vi "首页.vi"() -> ()   [LabVIEW 2016]
uses:
  <vilib>/Utility/miscctls.llb/LVPointTypeDef.ctl
  <vilib>/Utility/sysdir.llb/System Directory Type.ctl
  <vilib>/addons/database/_DB Variant To Data/Database Variant To Data.xnode
  PLC/PLC.lvlib
panel:
  out "小项目框 6":T1(xcontrol)
  out "小项目框 5":T1(xcontrol)
  out "小项目框":T1(xcontrol)
  out "湿度":string="75.5 %"
  out "室温":string="25.8 ℃"
  out "小项目框 4":T1(xcontrol)
  out "小项目框 3":T1(xcontrol)
  out "小项目框 2":T1(xcontrol)
  # "湿度:"
  # "室温:"
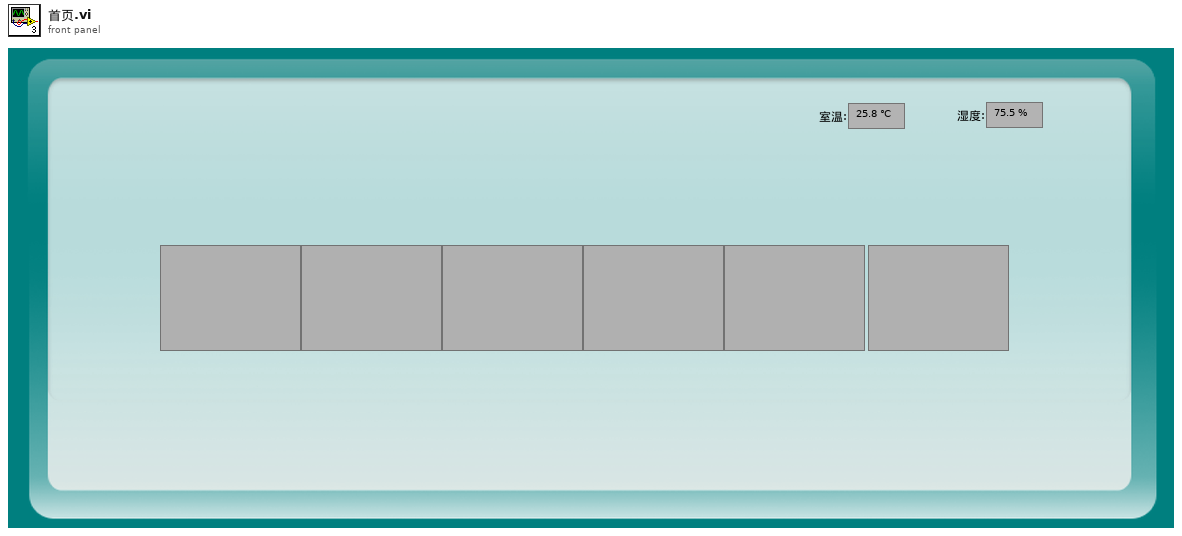
[diagram p1: front panel]
types:
  T1 = cluster{"中文项目名称":string, "英文项目名称":string, "单位":string, "浓度值":sgl}
  T2 = typedef "System Directory Type.ctl" = i32
  T3 = typedef "LVPointTypeDef.ctl" = cluster{"Horizontal":i16, "Vertical":i16}
  T4 = cluster{"AD0":sgl, "AD1":sgl, "AD2":sgl, "AD3":sgl, "AD4":sgl, "AD5":sgl}
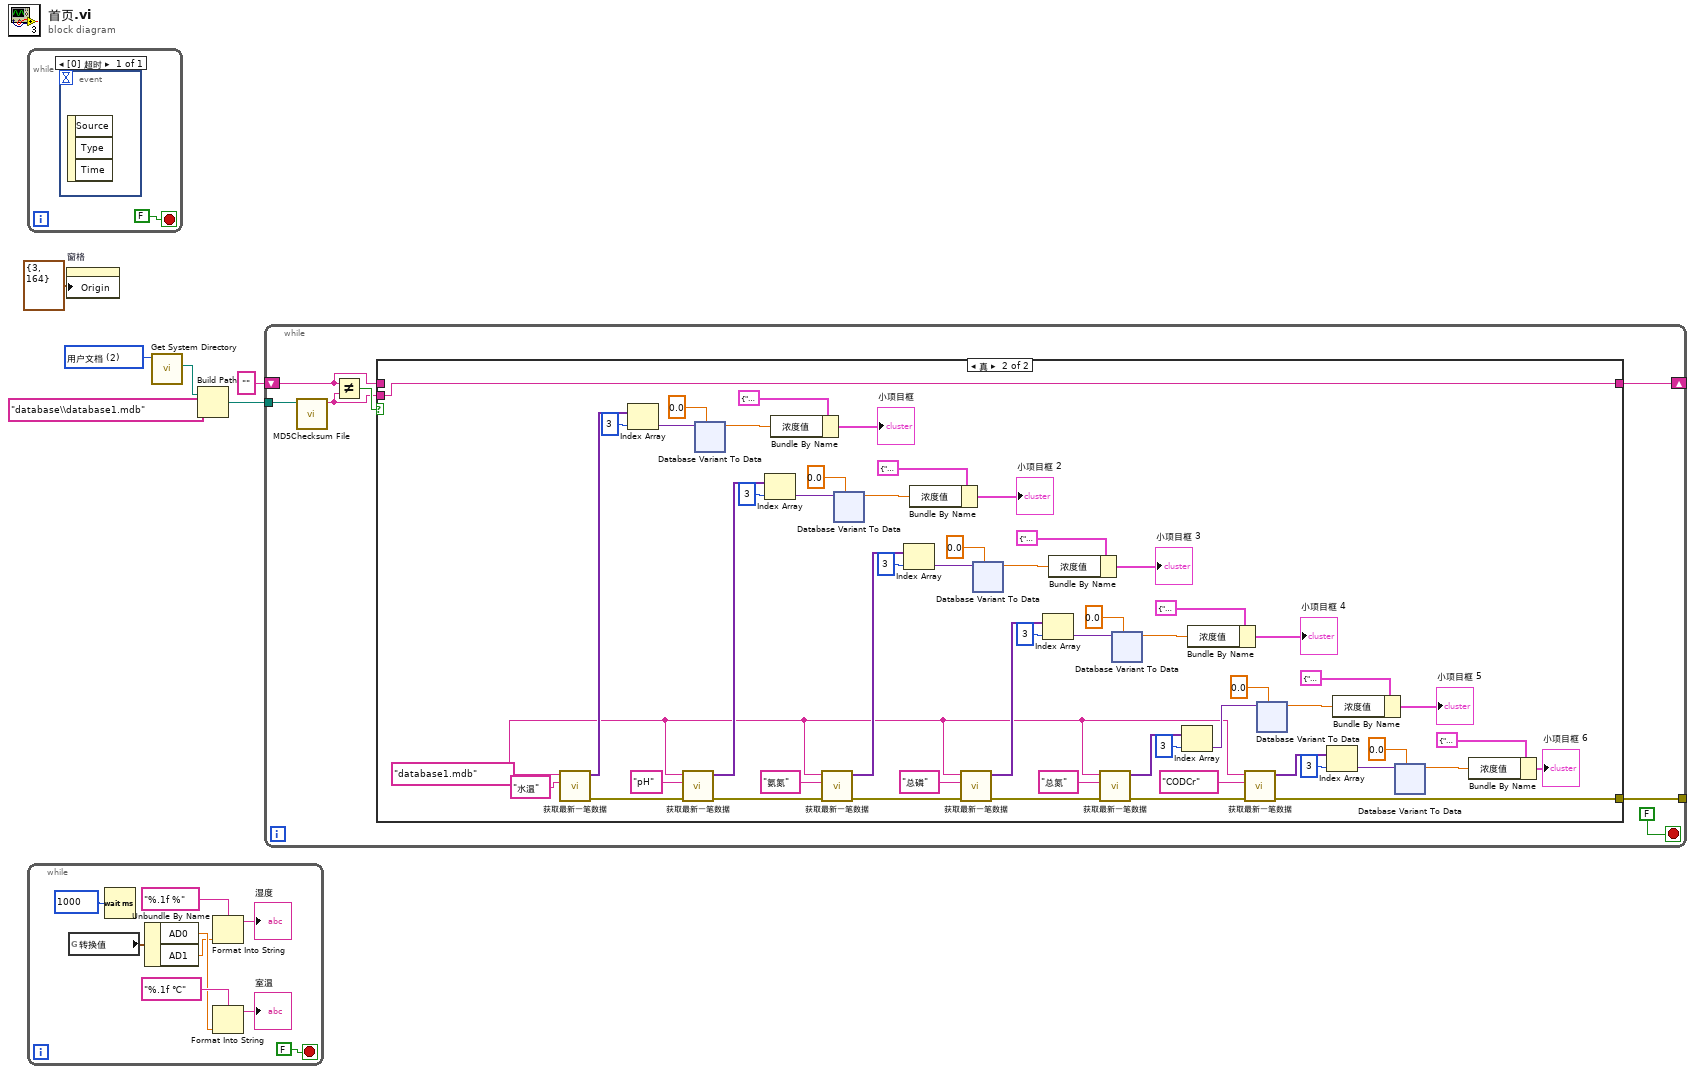
[diagram p0: block diagram]
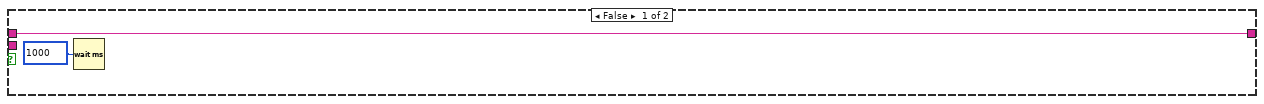
[diagram p2: hidden frame]
diagram:
  w5 = T2 2 items=["用户目录"=0, "用户桌面"=1, "用户文档"=2, "用户应用程序数据"=3, "用户设置"=4, "用户临时目录"=5, "公共文档"=6, "公共应用程序数据"=7, "公共设置"=8, "公共缓存"=13, "系统核心库"=9, "系统安装库"=10, "应用程序文件"=11, "启动盘根目录"=12] ("system directory type")
  n1 = while {
    stop <- FALSE stop-if-true
    n2 = event shown="[0] 超时" {
      selector: _ -> [_]
      dyn-events: _ -> [_]
      timeout: _ -> [_]
      event Timeout {
        n3 = event-data() -> ()  [unwired: 1 in, 3 out]
      }
    }
  }
  n4 = while {
    stop <- FALSE stop-if-true
    n5 = global read "采配水全局变量.vi" "转换值"() -> (w14:T4)
    n6 = Wait (ms)(milliseconds to wait=u32 1000 ("等待时间（毫秒）")) -> ()  [unwired: 1 out]
    n7 = Unbundle By Name(w14) -> ("AD0"=w9:sgl, "AD1"=w8:sgl)
    n8 = Format Into String(format string="%.1f %" ("格式字符串"), w8) -> (resulting string=→"湿度":string)  [unwired: 2 in, 1 out]
    n9 = Format Into String(format string="%.1f ℃" ("格式字符串"), w9) -> (resulting string=→"室温":string)  [unwired: 2 in, 1 out]
  }
  n10 = property on="窗格" class="Pane"("Origin"=T3 {"Horizontal"=3, "Vertical"=164} ("原点")) -> ()  [unwired: 2 in, 2 out]
  n11 = call <vilib>:"Get System Directory.vi"("system directory type"=w5) -> ("system directory"=w4:path)  [unwired: 10 in]
  n12 = Build Path(base path=w4, name or relative path="database\\database1.mdb" ("名称或相对路径")) -> (appended path=w2:path)
  n13 = while {
    tunnel: w2 -> [w23]
    shift-right: [w20] -> _
    shift-left: "" ("MD5 message-digest") -> [w19]
    tunnel: [w17] -> _
    stop <- FALSE stop-if-true
    n14 = call <vilib>:"MD5Checksum File.vi"("Path"=w23) -> ("MD5 message-digest"=w21:string)  [unwired: 9 in, 1 out]
    n15 = Not Equal?(x=w19, y=w21) -> (x != y?=w22:bool)
    n16 = case shown="真" w22 {
      tunnel: w21 -> [_ w81]
      tunnel: [w25 w81] -> w20
      tunnel: w19 -> [w25 _]
      tunnel: [_ w26] -> w17
      frame False {
        n17 = Wait (ms)(milliseconds to wait=u32 1000 ("等待时间（毫秒）")) -> ()  [unwired: 1 out]
      }
      frame True {
        w28 = "database1.mdb" ("名称或相对路径")
        n18 = call "获取最新一笔数据.vi"("table"="水温", "database"=w28) -> ("error out"=w49:errorcluster, "子数组"=w42:variant[])  [unwired: 8 in]
        n19 = Index Array(array=w42, index=3 ("索引")) -> (element=w45:variant)
        n20 = call "获取最新一笔数据.vi"("error in (no error)"=w49, "table"="pH", "database"=w28) -> ("error out"=w48:errorcluster, "子数组"=w70:variant[])  [unwired: 7 in]
        n21 = xnode "Database Variant To Data"("database variant"=w45, "type"=0.0) -> ("data"=w47:dbl)  [unwired: 1 in, 1 out]
        n22 = Index Array(array=w70, index=3 ("索引")) -> (element=w57:variant)
        n23 = Bundle By Name(cluster=T1 {"中文项目名称"="水温", "英文项目名称"="T", "单位"="℃", "浓度值"=0.0} ("小项目框 9"), "浓度值"=w47) -> (→"小项目框":T1)
        n24 = call "获取最新一笔数据.vi"("error in (no error)"=w48, "table"="氨氮", "database"=w28) -> ("error out"=w79:errorcluster, "子数组"=w67:variant[])  [unwired: 7 in]
        n25 = xnode "Database Variant To Data"("database variant"=w57, "type"=0.0) -> ("data"=w55:dbl)  [unwired: 1 in, 1 out]
        n26 = Index Array(array=w67, index=3 ("索引")) -> (element=w63:variant)
        n27 = Bundle By Name(cluster=T1 {"中文项目名称"="酸碱度", "英文项目名称"="pH", "单位"="", "浓度值"=0.0} ("小项目框 9"), "浓度值"=w55) -> (→"小项目框 2":T1)
        n28 = call "获取最新一笔数据.vi"("error in (no error)"=w79, "table"="总磷", "database"=w28) -> ("error out"=w51:errorcluster, "子数组"=w64:variant[])  [unwired: 7 in]
        n29 = xnode "Database Variant To Data"("database variant"=w63, "type"=0.0) -> ("data"=w61:dbl)  [unwired: 1 in, 1 out]
        n30 = Index Array(array=w64, index=3 ("索引")) -> (element=w60:variant)
        n31 = Bundle By Name(cluster=T1 {"中文项目名称"="氨氮", "英文项目名称"="NH3-N", "单位"="mg/L", "浓度值"=0.0} ("小项目框 9"), "浓度值"=w61) -> (→"小项目框 3":T1)
        n32 = call "获取最新一笔数据.vi"("error in (no error)"=w51, "table"="总氮", "database"=w28) -> ("error out"=w30:errorcluster, "子数组"=w73:variant[])  [unwired: 7 in]
        n33 = xnode "Database Variant To Data"("database variant"=w60, "type"=0.0) -> ("data"=w58:dbl)  [unwired: 1 in, 1 out]
        n34 = Index Array(array=w73, index=3 ("索引")) -> (element=w54:variant)
        n35 = Bundle By Name(cluster=T1 {"中文项目名称"="总磷", "英文项目名称"="TP", "单位"="mg/L", "浓度值"=0.0} ("小项目框 9"), "浓度值"=w58) -> (→"小项目框 4":T1)
        n36 = call "获取最新一笔数据.vi"("error in (no error)"=w30, "table"="CODCr", "database"=w28) -> ("error out"=w26:errorcluster, "子数组"=w29:variant[])  [unwired: 7 in]
        n37 = xnode "Database Variant To Data"("database variant"=w54, "type"=0.0) -> ("data"=w52:dbl)  [unwired: 1 in, 1 out]
        n38 = Index Array(array=w29, index=3 ("索引")) -> (element=w34:variant)
        n39 = Bundle By Name(cluster=T1 {"中文项目名称"="总氮", "英文项目名称"="TN", "单位"="mg/L", "浓度值"=0.0} ("小项目框 9"), "浓度值"=w52) -> (→"小项目框 5":T1)
        n40 = xnode "Database Variant To Data"("database variant"=w34, "type"=0.0) -> ("data"=w36:dbl)  [unwired: 1 in, 1 out]
        n41 = Bundle By Name(cluster=T1 {"中文项目名称"="化学需氧量", "英文项目名称"="CODcr", "单位"="mg/L", "浓度值"=0.0} ("小项目框 9"), "浓度值"=w36) -> (→"小项目框 6":T1)
      }
    }
  }
